vi "crane_pressure_view_RecurDyn.vi"() -> ()   [LabVIEW 2020]
panel:
  out "l5_ground_pressure":dbl(slide)
  out "l4_ground_pressure":dbl(slide)
  out "l3_ground_pressure":dbl(slide)
  out "l2_ground_pressure":dbl(slide)
  out "l1_ground_pressure":dbl(slide)
  out "error out":errorcluster
  in  "stop":bool
  out "period(Hz)":dbl(knob) scale=0.0..10.0
  out "l5_gp_max":bool
  out "l4_gp_max":bool
  out "l3_gp_max":bool
  out "l2_gp_max":bool
  out "l1_gp_max":bool
  out "r5_gp_max":bool
  out "r4_gp_max":bool
  out "r3_gp_max":bool
  out "r2_gp_max":bool
  out "r1_gp_max":bool
  out "MaxGroundPressure":T1(graph)
  out "Load_state":dbl(graph)
  out "Angle":T2(graph)
  in  "Load(ton)":dbl(slide) scale=40.0..120.0
  in  "boom_angle(degree)":dbl(knob) scale=40.0..70.0
  in  "swing_angle(degree)":dbl(knob) scale=0.0..180.0
  out "r5_ground_pressure":dbl(slide) scale=0.0..500000.0
  out "r4_ground_pressure":dbl(slide) scale=0.0..500000.0
  out "r3_ground_pressure":dbl(slide) scale=0.0..500000.0
  out "r2_ground_pressure":dbl(slide) scale=0.0..500000.0
  out "r1_ground_pressure":dbl(slide) scale=0.0..500000.0
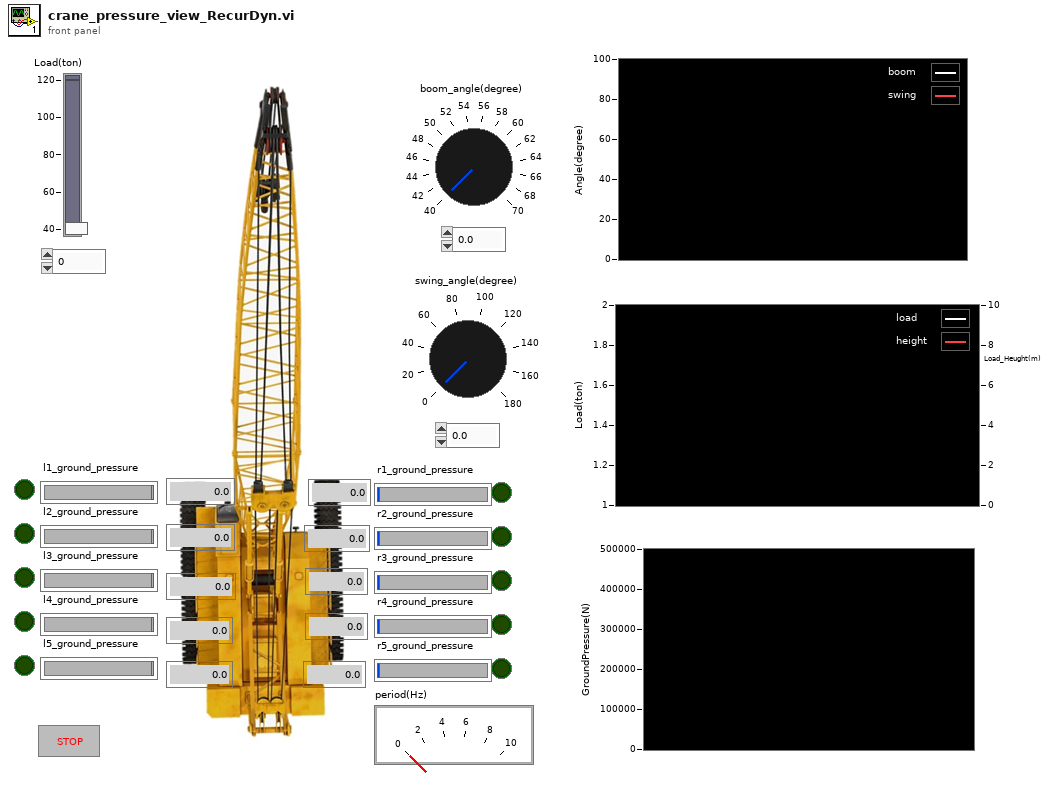
[diagram p1: front panel]
types:
  T1 = cluster{dbl, dbl, dbl, dbl, dbl, dbl, dbl, dbl, dbl, dbl}
  T2 = cluster{"boom_angle(degree)":dbl, "swing_angle(degree)":dbl}
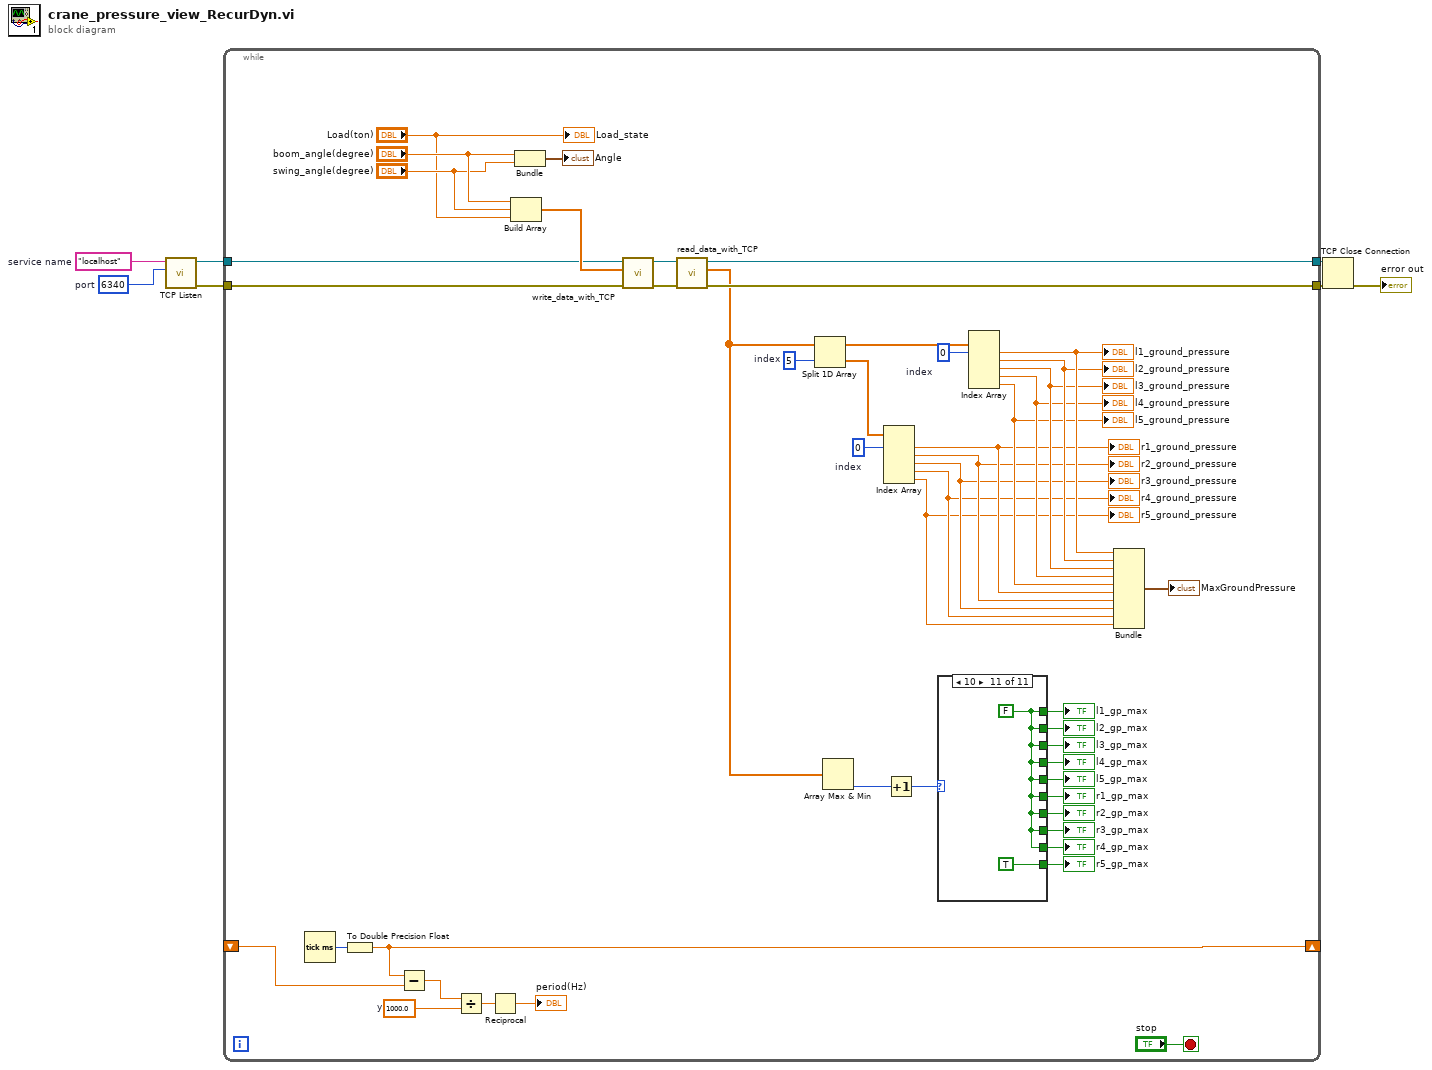
[diagram p0: block diagram]
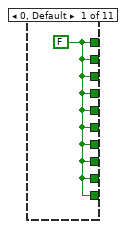
[diagram p2: hidden frame]
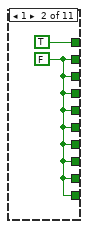
[diagram p3: hidden frame]
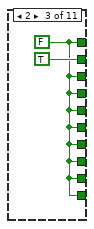
[diagram p4: hidden frame]
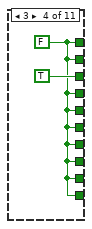
[diagram p5: hidden frame]
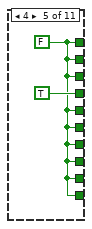
[diagram p6: hidden frame]
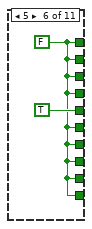
[diagram p7: hidden frame]
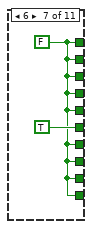
[diagram p8: hidden frame]
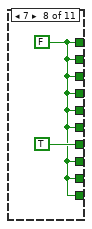
[diagram p9: hidden frame]
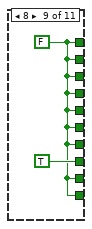
[diagram p10: hidden frame]
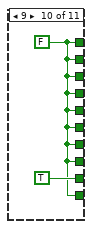
[diagram p11: hidden frame]
diagram:
  w6 = u16 6340  # port
  w7 = "localhost"  # service name
  n1 = call <vilib>:"TCP Listen.vi"("port"=w6, "service name"=w7) -> ("error out"=w4:errorcluster, "connection ID"=w5:refnum<k5>)  [unwired: 5 in, 3 out]
  n2 = while {
    tunnel: w5 -> [w39]
    tunnel: w4 -> [w38]
    tunnel: [w37] -> w3
    tunnel: [w36] -> w2
    shift-right: [w31] -> _
    shift-left: _ -> [w30]
    stop <- "stop" stop-if-true
    w25 = 0  # index
    w27 = 5  # index
    w34 = 1000.0  # y
    w40 = 0  # index
    n3 = Tick Count (ms)() -> (millisecond timer value=w32:u32)
    n4 = To Double Precision Float(number=w32) -> (double precision float=w31:dbl)
    n5 = Subtract(x=w31, y=w30) -> (x-y=w35:dbl)
    n6 = Divide(x=w35, y=w34) -> (x/y=w33:dbl)
    n7 = Reciprocal(x=w33) -> (1/x=→"period(Hz)":dbl)
    n8 = Build Array("boom_angle(degree)", "swing_angle(degree)", "Load(ton)") -> (w44:dbl[])
    n9 = Bundle("boom_angle(degree)"="boom_angle(degree)", "swing_angle(degree)"="swing_angle(degree)") -> (→"Angle":T2)  [unwired: 1 in]
    n10 = call "write_data_with_TCP.vi"("error_in"=w38, "data_in"=w44, "TCP_ref_in"=w39) -> ("error_out"=w41:errorcluster, "TCP_ref_out"=w42:refnum<k5>)  [unwired: 7 in]
    n11 = call "read_data_with_TCP.vi"("error_in"=w41, "TCP_ref_in"=w42) -> ("error_out"=w36:errorcluster, "data_out"=w20:dbl[], "TCP_ref_out"=w37:refnum<k5>)  [unwired: 7 in]
    n12 = Split 1D Array(array=w20, index=w27) -> (first subarray=w24:dbl[], second subarray=w26:dbl[])
    n13 = Array Max & Min(array=w20) -> (min index (indices)=w8:i32)  [unwired: 3 out]
    n14 = Index Array(array=w26, index #1=w25) -> (element #1=w14:dbl, element #2=w13:dbl, element #3=w12:dbl, element #4=w11:dbl, element #5=w10:dbl)  [unwired: 4 in]
    "r1_ground_pressure" <- w14
    "r2_ground_pressure" <- w13
    "r3_ground_pressure" <- w12
    "r4_ground_pressure" <- w11
    "r5_ground_pressure" <- w10
    n15 = Increment(x=w8) -> (x+1=w45:i32)
    n16 = case shown="10" w45 {
      tunnel: [w56 TRUE w59 w61 w63 w65 w67 w69 w71 w73 w75] -> w55
      tunnel: [w56 w57 TRUE w61 w63 w65 w67 w69 w71 w73 w75] -> w54
      tunnel: [w56 w57 w59 TRUE w63 w65 w67 w69 w71 w73 w75] -> w53
      tunnel: [w56 w57 w59 w61 TRUE w65 w67 w69 w71 w73 w75] -> w52
      tunnel: [w56 w57 w59 w61 w63 TRUE w67 w69 w71 w73 w75] -> w51
      tunnel: [w56 w57 w59 w61 w63 w65 TRUE w69 w71 w73 w75] -> w50
      tunnel: [w56 w57 w59 w61 w63 w65 w67 TRUE w71 w73 w75] -> w49
      tunnel: [w56 w57 w59 w61 w63 w65 w67 w69 TRUE w73 w75] -> w48
      tunnel: [w56 w57 w59 w61 w63 w65 w67 w69 w71 TRUE w75] -> w47
      tunnel: [w56 w57 w59 w61 w63 w65 w67 w69 w71 w73 TRUE] -> w46
      frame 0, Default {
        w56 = FALSE
      }
      frame 1 {
        w57 = FALSE
      }
      frame 2 {
        w59 = FALSE
      }
      frame 3 {
        w61 = FALSE
      }
      frame 4 {
        w63 = FALSE
      }
      frame 5 {
        w65 = FALSE
      }
      frame 6 {
        w67 = FALSE
      }
      frame 7 {
        w69 = FALSE
      }
      frame 8 {
        w71 = FALSE
      }
      frame 9 {
        w73 = FALSE
      }
      frame 10 {
        w75 = FALSE
      }
    }
    "r1_gp_max" <- w50
    "r2_gp_max" <- w49
    "r3_gp_max" <- w48
    "r4_gp_max" <- w47
    "r5_gp_max" <- w46
    "l1_gp_max" <- w55
    "l2_gp_max" <- w54
    "l3_gp_max" <- w53
    "l4_gp_max" <- w52
    "l5_gp_max" <- w51
    n17 = Index Array(array=w24, index #1=w40) -> (element #1=w19:dbl, element #2=w18:dbl, element #3=w17:dbl, element #4=w16:dbl, element #5=w15:dbl)  [unwired: 4 in]
    "l1_ground_pressure" <- w19
    "l2_ground_pressure" <- w18
    "l3_ground_pressure" <- w17
    "l4_ground_pressure" <- w16
    "l5_ground_pressure" <- w15
    n18 = Bundle(w19, w18, w17, w16, w15, w14, w13, w12, w11, w10) -> (→"MaxGroundPressure":T1)  [unwired: 1 in]
    "Load_state" <- "Load(ton)"
  }
  n19 = TCP Close Connection(connection ID=w3, error in (no error)=w2) -> (error out=→"error out":errorcluster)  [unwired: 1 in, 1 out]
